vi "_PC_Pub_Read_Spreadsheet.vi"(7 "format (%s)":string="%s", 8 "error in (no error)":errorcluster, 10 "number of rows (all:-1)":i32=-1, 11 "file path (dialog if empty)":path) -> (0 "error out":errorcluster, 1 "first row":string[](array[string]), 2 "all rows":string[][](array[string]), 3 "new file path (Not A Path if cancelled)":path)   [LabVIEW 2018]
panel:
  out "EOF?":bool
  in  "delimiter (\\t)":string="\t"
  in  "type (empty)":string[][](array[string])
  in  "transpose? (F)":bool
  out "mark after read (chars.)":i32
  in  "max characters/row  (no limit:0)":i32
  in  "start of read offset (chars.:0)":i32
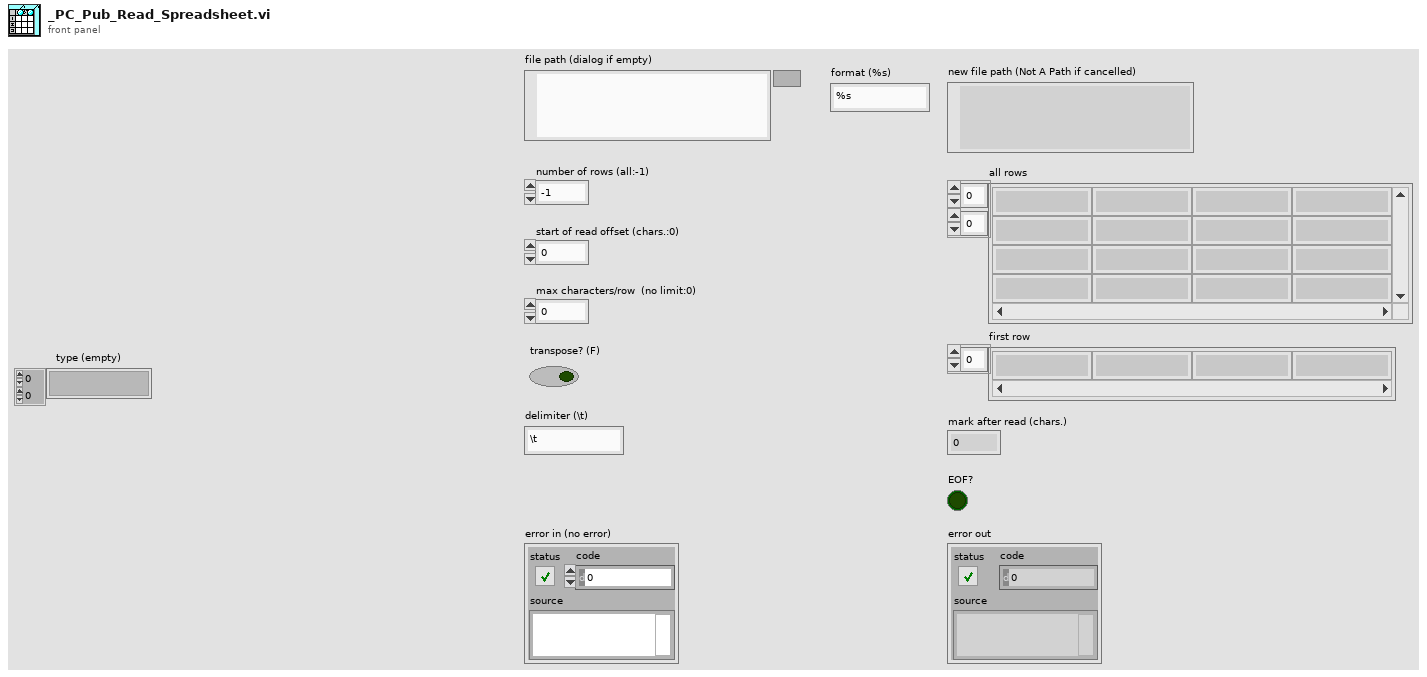
[diagram p1: front panel]
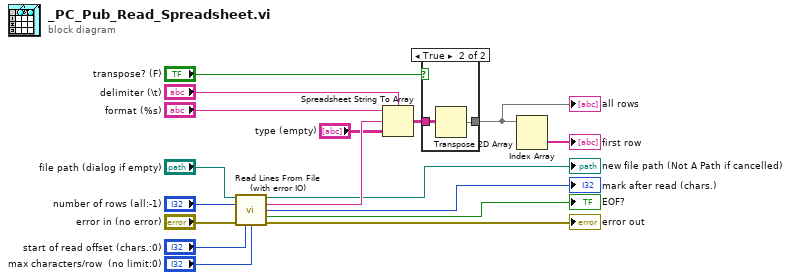
[diagram p0: block diagram]
diagram:
  n1 = call <vilib>:"Read Lines From File (with error IO).vi"("file path (dialog if empty)"="file path (dialog if empty)", "number of rows (all:-1)"="number of rows (all:-1)", "error in (no error)"="error in (no error)", "start of read offset (chars.:0)"="start of read offset (chars.:0)", "max characters/row  (no limit:0)"="max characters/row  (no limit:0)") -> ("new file path (Not A Path if cancelled)"=→"new file path (Not A Path if cancelled)":path, "line string"=w13:string, "mark after read (chars.)"=→"mark after read (chars.)":i32, "EOF?"=→"EOF?":bool, "error out"=→"error out":errorcluster)  [unwired: 6 in]
  n2 = Spreadsheet String To Array(delimiter (Tab)="delimiter (\\t)", format string="format (%s)", spreadsheet string=w13, array type (2D Dbl)="type (empty)") -> (array=w5:string[][])
  n3 = case shown="True" "transpose? (F)" {
    tunnel: w5 -> [w18 w20]
    tunnel: [w18 w19] -> w3
    frame False {
    }
    frame True {
      n4 = Transpose 2D Array(2D array=w20) -> (transposed array=w19:string[][])
    }
  }
  "all rows" <- w3
  n5 = Index Array(array=w3) -> (element=→"first row":string[])  [unwired: 2 in]
